vi "CompileCalibration.vi"(8 "error in":errorcluster, 9 "Compiler Settings":T2={"Python Path"=path "", "Main File"="makesequence.py", "Meta File"="makesequence.py", "Aux File"="makesequence.py", "Pre File"="metascript.txt"}) -> (0 "error out":errorcluster, 1 "Compiler Settings 2":T2={"Python Path"=path "", "Main File"="makesequence.py", "Meta File"="makesequence.py", "Aux File"="makesequence.py", "Pre File"="metascript.txt"}, 3 "Exp out":T1(array[cluster]))   [LabVIEW 2019]
uses:
  PulseCompiler/CompilerSettings.ctl
  <vilib>/regexp/Match Regular Expression.xnode
panel:
  out "Array":string[](array[string])
  in  "stop":bool
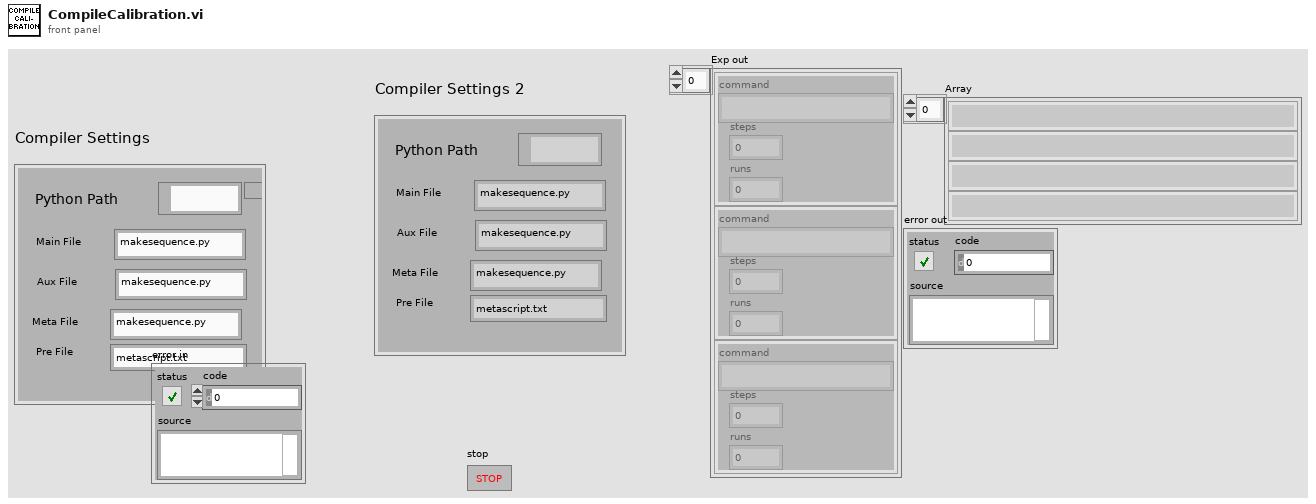
[diagram p1: front panel]
types:
  T1 = cluster{"command":string, "steps":i32, "runs":i32}[]
  T2 = typedef "CompilerSettings.ctl" = cluster{"Python Path":path, "Main File":string, "Meta File":string, "Aux File":string, "Pre File":string}
  T3 = enum16{"open", "replace", "create", "open or create", "replace or create", "replace or create with confirmation"}
  T4 = cluster{"command":string, "steps":i32, "runs":i32}
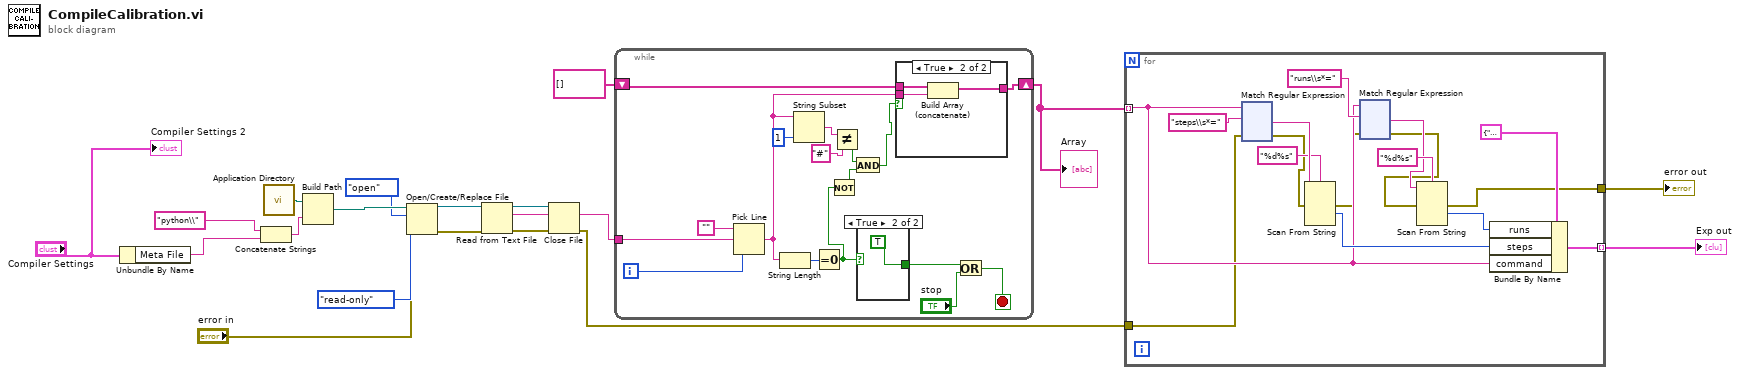
[diagram p0: block diagram]
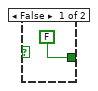
[diagram p3: hidden frame]
diagram:
  n1 = Unbundle By Name("Compiler Settings") -> ("Meta File"=w15:string)
  n2 = Concatenate Strings("python\\" ("name or relative path"), w15) -> (w17:string)
  n3 = call <vilib>:"Application Directory.vi"() -> ("Application Directory"=w19:path)
  n4 = Build Path(base path=w19, name or relative path=w17) -> (appended path=w18:path)
  n5 = Open/Create/Replace File(file path (use dialog)=w18, error in="error in", operation (0:open)=T3."open", access (0:read/write)=enum16{"read/write", "read-only", "write-only"}."read-only") -> (refnum out=w11:refnum<file>, error out=w12:errorcluster)  [unwired: 2 in, 1 out]
  n6 = Read from Text File(file (use dialog)=w11, error in=w12) -> (refnum out=w5:refnum<file>, text=w9:string, error out=w4:errorcluster)  [unwired: 2 in, 1 out]
  n7 = Close File(refnum=w5, error in=w4) -> (error out=w2:errorcluster)  [unwired: 1 out]
  n8 = while {
    shift-right: [w34] -> w7
    shift-left: string[] [] -> [w35]
    tunnel: w9 -> [w28]
    i -> [w36]
    stop <- w29 stop-if-true
    n9 = Pick Line(string ("")="", multi-line string=w28, line index=w36) -> (output string=w25:string)
    n10 = String Length(string=w25) -> (length=w32:i32)
    n11 = String Subset(string=w25, length (rest)=1 ("length (rest)")) -> (substring=w26:string)  [unwired: 1 in]
    n12 = Equal To 0?(x=w32) -> (x = 0?=w23:bool)
    n13 = Not(x=w23) -> (.not. x?=w20:bool)
    n14 = Not Equal?(x=w26, y="#") -> (x != y?=w21:bool)
    n15 = And(x=w21, y=w20) -> (x .and. y?=w22:bool)
    n16 = case shown="True" w23 {
      tunnel: [FALSE TRUE] -> w31
      frame False {
      }
      frame True {
      }
    }
    n17 = case shown="True" w22 {
      tunnel: w35 -> [w37 w40]
      tunnel: [w37 w39] -> w34
      tunnel: w25 -> [_ w38]
      frame False {
      }
      frame True {
        n18 = Build Array (concatenate)(w40, w38) -> (w39:string[])
      }
    }
    n19 = Or(x=w31, y="stop") -> (x .or. y?=w29:bool)
  }
  "Array" <- w7
  n20 = for {
    tunnel: w7 -> [w48] mode=indexing
    tunnel: [w49] -> w6 mode=indexing
    tunnel: w2 -> [w47]
    tunnel: [w43] -> w1
    n21 = xnode "Match Regular Expression"("input string"=w48, "regular expression"="steps\\s*=", "error in"=w47) -> ("after match"=w56:string, "error out"=w46:errorcluster)  [unwired: 3 in, 3 out]
    n22 = Scan From String(format string="%d%s", input string=w56, error in=w46) -> (error out=w45:errorcluster, output 1=w50:i32)  [unwired: 4 in, 2 out]
    n23 = xnode "Match Regular Expression"("input string"=w48, "regular expression"="runs\\s*=", "error in"=w45) -> ("after match"=w53:string, "error out"=w44:errorcluster)  [unwired: 3 in, 3 out]
    n24 = Scan From String(format string="%d%s", input string=w53, error in=w44) -> (error out=w43:errorcluster, output 1=w51:i32)  [unwired: 4 in, 2 out]
    n25 = Bundle By Name(cluster=T4 {"command"="", "steps"=0, "runs"=0}, "runs"=w51, "steps"=w50, "command"=w48) -> (w49:T4)
  }
  "Exp out" <- w6
  "error out" <- w1
  "Compiler Settings 2" <- "Compiler Settings"
